vi "XYWavenameLengthDialog.vi"() -> (0 "Boolean 2":bool)   [LabVIEW 2016, in "LVtoITX.lvclass"]
uses:
  LVtoITX.lvclass
panel:
  in  "Boolean":bool
  # "Your wavename is too long for Igor!\nYour filename should be 25 characters or less!\nTry again!"
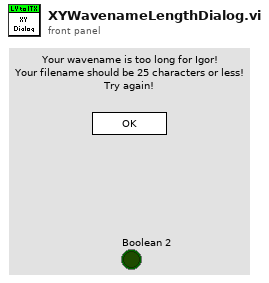
[diagram p1: front panel]
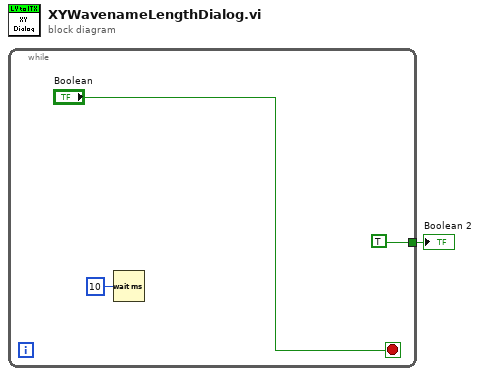
[diagram p0: block diagram]
diagram:
  n1 = while {
    tunnel: [TRUE ("Boolean 2")] -> w1
    stop <- "Boolean" stop-if-true
    n2 = Wait (ms)(milliseconds to wait=u32 10) -> ()  [unwired: 1 out]
  }
  "Boolean 2" <- w1
